vi "MWT_labview_final2.vi"() -> ()   [LabVIEW 2019]
uses:
  <vilib>/BLE/type_def/connection_status_bundle.ctl
  <vilib>/BLE/type_def/address_type.ctl
  <vilib>/BLE/ble_functions/ble_write_by_service_characteristic_uint8array.vi
panel:
  out "Omega0":dbl(graph)
  out "Omega0":dbl
  out "characteristic value":u8[](array[numeric])
  in  "transmission inteveral (Seconds)":u8[](array[numeric]) format="%02x"
  out "Omega4":dbl(graph)
  out "Omega4":dbl
  out "Omega1":dbl(graph)
  out "Omega1":dbl
  out "Omega3":dbl(graph)
  out "Omega3":dbl
  in  "stop":bool
  out "Reading data":bool
  out "Connected":bool
  out "Device Name":string
  out "Handle table":string[][](array[string])
  out "Connection Status":T1={"MAC Address"="", "cnx handle"=0, "cnx flags"=0, "Address Type"=125, "Connection Interval (ms)"=125, "Timeout(ms)"=125, "Latency"=0, "bonding handle"=0} {"Address Type" items=["Public", "Random"]}
  out "Scanning":bool
  in  "COM Bluegiga in":refnum<visa-resource-name>="COM13"
  out "Devices":string[][](array[string])
  out "BLED112 Dongle Info":string
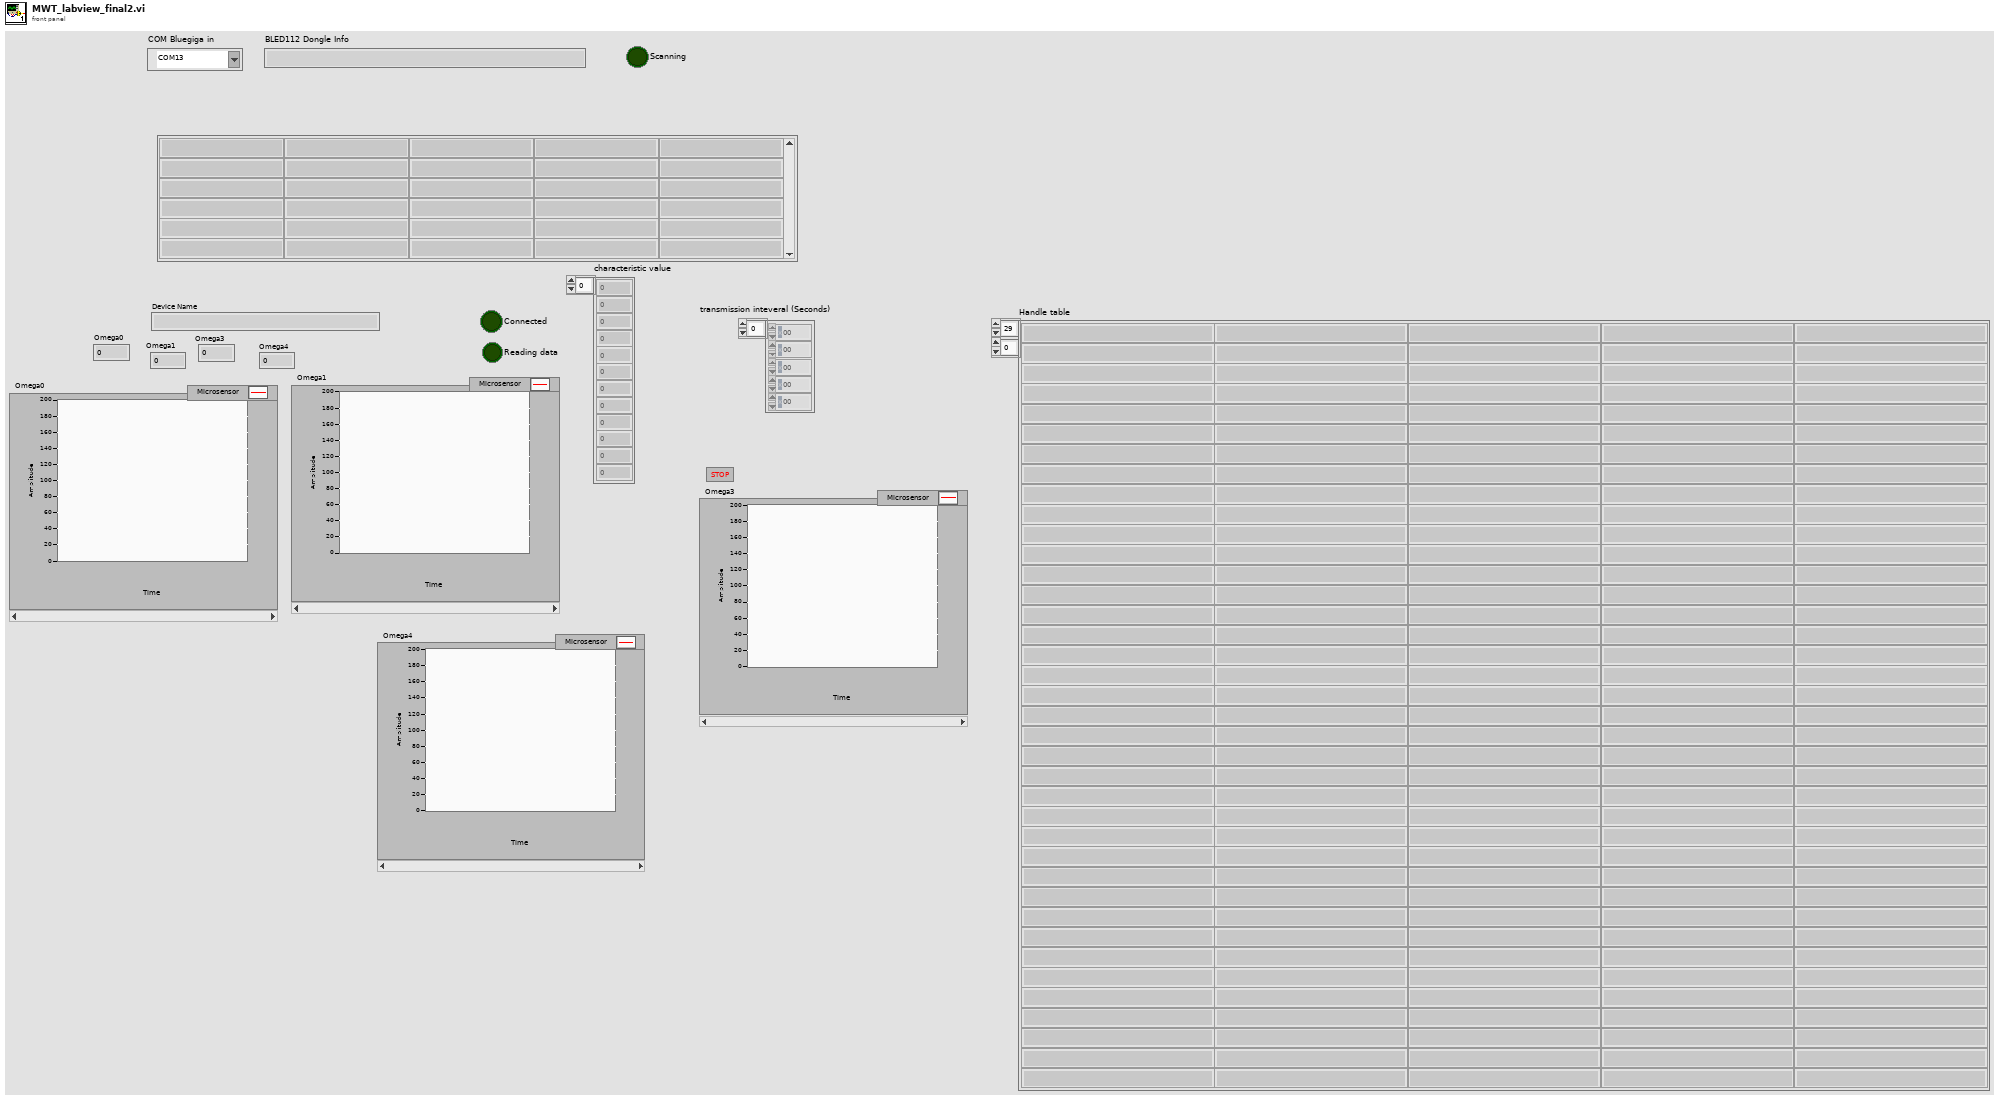
[diagram p1: front panel]
types:
  T1 = typedef "connection_status_bundle.ctl" = cluster{"MAC Address":string, "cnx handle":u8, "cnx flags":u8, "Address Type":T2, "Connection Interval (ms)":u16, "Timeout(ms)":u16, "Latency":u16, "bonding handle":u8}
  T2 = typedef "address_type.ctl" = u8
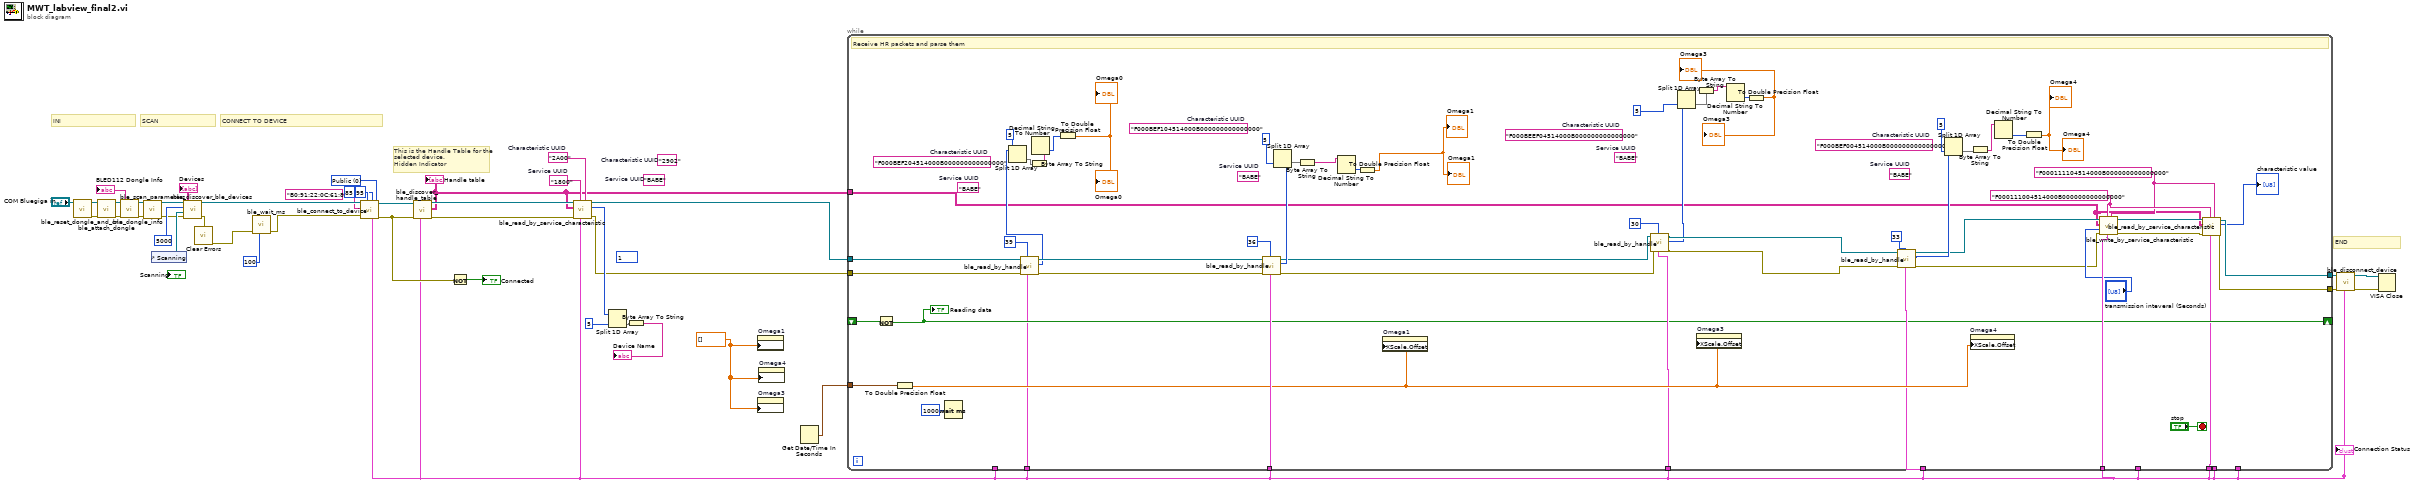
[diagram p0: block diagram]
diagram:
  w14 = T2 0 items=["Public", "Random"] ("Address Type")
  w12 = dbl[] [] ("History Data")
  (unwired) "2902"  # Characteristic UUID
  (unwired) "BABE"  # Service UUID
  (unwired) u16 1 ("Value(16bit)")
  w21 = "2A00"  # Characteristic UUID
  w22 = "1800"  # Service UUID
  # "END"
  # "This is the Handle Table for the\nselected device. \nHidden Indicator"
  # "CONNECT TO DEVICE"
  # "SCAN"
  # "INI"
  n1 = call <vilib>:"ble_reset_dongle_and_cnx.vi"("COM Bluegiga in"="COM Bluegiga in") -> ("error out"=w33:errorcluster, "COM Bluegiga out"=w31:refnum<visa-resource-name>)  [unwired: 9 in]
  n2 = call <vilib>:"ble_attach_dongle.vi"("error in (no error)"=w33, "COM Bluegiga in"=w31) -> ("error out"=w35:errorcluster, "COM Bluegiga out"=w34:refnum<visa-resource-name>)  [unwired: 8 in]
  n3 = call <vilib>:"ble_dongle_info.vi"("error in (no error)"=w35, "COM Bluegiga in"=w34) -> ("error out"=w38:errorcluster, "info"=→"BLED112 Dongle Info":string, "COM Bluegiga out"=w39:refnum<visa-resource-name>)  [unwired: 7 in]
  n4 = call <vilib>:"ble_scan_parameters.vi"("error in (no error)"=w38, "COM Bluegiga in"=w39) -> ("error out"=w36:errorcluster, "COM Bluegiga out"=w37:refnum<visa-resource-name>)  [unwired: 7 in, 1 out]
  n5 = control-ref of="Scanning"() -> (w40:refnum<vi>)
  n6 = call <vilib>:"ble_discover_ble_devices.vi"("error in (no error)"=w36, "LED ref"=w40, "Scan Duration (10000ms)"=u32 5000, "COM Bluegiga in"=w37) -> ("error out"=w29:errorcluster, "Devices"=→"Devices":string[][], "COM Bluegiga out"=w15:refnum<visa-resource-name>)  [unwired: 5 in]
  n7 = call <vilib>:"Clear Errors.vi"("error in (no error)"=w29) -> ("error out"=w18:errorcluster)  [unwired: 5 in, 1 out]
  n8 = call <vilib>:"ble_wait_ms.vi"("milliseconds to wait (100)"=u32 100, "error in (no error)"=w18) -> ("error out"=w17:errorcluster)  [unwired: 9 in]
  n9 = call <vilib>:"ble_connect_to_device.vi"("Address Type"=w14, "Connection Interval Max (95ms)"=u16 95, "Connection Interval Min (75ms)"=u16 85, "error in (no error)"=w17, "MAC Address"="B0:91:22:0C:61:84", "COM Bluegiga in"=w15) -> ("error out"=w23:errorcluster, "COM Bluegiga out"=w30:refnum<visa-resource-name>, "Connection Status"=w2:T1)  [unwired: 3 in]
  "Connection Status" <- w2
  n10 = call <vilib>:"ble_discover_handle_table.vi"("Connection Status"=w2, "error in (no error)"=w23, "COM Bluegiga in"=w30) -> ("error out"=w28:errorcluster, "Handle table"=w1:string[][], "COM Bluegiga out"=w27:refnum<visa-resource-name>)  [unwired: 6 in]
  "Handle table" <- w1
  n11 = Not(x=w23) -> (.not. x?=→"Connected":bool)
  n12 = call <vilib>:"ble_read_by_service_characteristic.vi"("Characteristic UUID"=w21, "Connection Status"=w2, "Service UUID"=w22, "error in (no error)"=w28, "Handle table"=w1, "COM Bluegiga in"=w27) -> ("error out"=w5:errorcluster, "characteristic value"=w20:u8[], "COM Bluegiga out"=w6:refnum<visa-resource-name>)  [unwired: 3 in]
  n13 = Split 1D Array(array=w20, index=5) -> (second subarray=w19:u8[])  [unwired: 1 out]
  n14 = Byte Array To String(unsigned byte array=w19) -> (string=→"Device Name":string)
  n15 = property on="Omega1" class="WFChart (strict)"("History Data"=w12) -> ()  [unwired: 2 in, 2 out]
  n16 = property on="Omega3" class="WFChart (strict)"("History Data"=w12) -> ()  [unwired: 2 in, 2 out]
  n17 = property on="Omega4" class="WFChart (strict)"("History Data"=w12) -> ()  [unwired: 2 in, 2 out]
  n18 = Get Date/Time In Seconds() -> (seconds since 1Jan1904=w9:timestamp)
  n19 = while {
    shift-right: [w72] -> _
    shift-left: _ -> [w101]
    tunnel: w2 -> [w76]
    tunnel: w2 -> [w92]
    tunnel: w2 -> [_]
    tunnel: w2 -> [w74]
    tunnel: w9 -> [w82]
    tunnel: w2 -> [_]
    tunnel: w2 -> [w80]
    tunnel: w6 -> [w68]
    tunnel: w5 -> [w67]
    tunnel: w2 -> [w66]
    tunnel: w2 -> [_]
    tunnel: w2 -> [_]
    tunnel: [w54] -> w4
    tunnel: [w53] -> w3
    tunnel: w2 -> [w49]
    tunnel: w1 -> [w48]
    stop <- "stop" stop-if-true
    w51 = "F000111004514000B000000000000000" ("Service UUID")
    w50 = "F000111104514000B000000000000000" ("Characteristic UUID")
    (unwired) "F000BEF004514000B000000000000000"  # Characteristic UUID
    (unwired) "BABE"  # Service UUID
    (unwired) "F000BEF204514000B000000000000000"  # Characteristic UUID
    (unwired) "BABE"  # Service UUID
    (unwired) "F000BEF104514000B000000000000000"  # Characteristic UUID
    (unwired) "BABE"  # Service UUID
    (unwired) "F000BEEF04514000B000000000000000"  # Characteristic UUID
    (unwired) "BABE"  # Service UUID
    # "Receive HR packets and parse them"
    n20 = Not(x=w101) -> (.not. x?=w72:bool)
    "Reading data" <- w72
    n21 = To Double Precision Float(number=w82) -> (double precision float=w83:dbl)
    n22 = Wait (ms)(milliseconds to wait=u32 1000) -> ()  [unwired: 1 out]
    n23 = call <vilib>:"ble_read_by_handle.vi"("Connection Status"=w66, "Handle"=u16 39, "error in (no error)"=w67, "COM Bluegiga in"=w68) -> ("error out"=w70:errorcluster, "characteristic value"=w65:u8[], "COM Bluegiga out"=w71:refnum<visa-resource-name>)  [unwired: 5 in]
    n24 = Split 1D Array(array=w65, index=5) -> (second subarray=w57:u8[])  [unwired: 1 out]
    n25 = Byte Array To String(unsigned byte array=w57) -> (string=w90:string)
    n26 = Decimal String To Number(string=w90) -> (number=w89:i32)  [unwired: 2 in, 1 out]
    n27 = To Double Precision Float(number=w89) -> (double precision float=→"Omega0" →"Omega0":dbl)
    n28 = call <vilib>:"ble_read_by_handle.vi"("Connection Status"=w92, "Handle"=u16 36, "error in (no error)"=w70, "COM Bluegiga in"=w71) -> ("error out"=w77:errorcluster, "characteristic value"=w93:u8[], "COM Bluegiga out"=w78:refnum<visa-resource-name>)  [unwired: 5 in]
    n29 = Split 1D Array(array=w93, index=5) -> (second subarray=w94:u8[])  [unwired: 1 out]
    n30 = Byte Array To String(unsigned byte array=w94) -> (string=w46:string)
    n31 = Decimal String To Number(string=w46) -> (number=w47:i32)  [unwired: 2 in, 1 out]
    n32 = To Double Precision Float(number=w47) -> (double precision float=→"Omega1" →"Omega1":dbl)
    n33 = property on="Omega1" class="WFChart (strict)"("XScale.Offset"=w83) -> ()  [unwired: 2 in, 2 out]
    n34 = call <vilib>:"ble_read_by_handle.vi"("Connection Status"=w76, "Handle"=u16 30, "error in (no error)"=w77, "COM Bluegiga in"=w78) -> ("error out"=w63:errorcluster, "characteristic value"=w62:u8[], "COM Bluegiga out"=w64:refnum<visa-resource-name>)  [unwired: 5 in]
    n35 = Split 1D Array(array=w62, index=5) -> (second subarray=w99:u8[])  [unwired: 1 out]
    n36 = property on="Omega3" class="WFChart (strict)"("XScale.Offset"=w83) -> ()  [unwired: 2 in, 2 out]
    n37 = Byte Array To String(unsigned byte array=w99) -> (string=w98:string)
    n38 = Decimal String To Number(string=w98) -> (number=w97:i32)  [unwired: 2 in, 1 out]
    n39 = To Double Precision Float(number=w97) -> (double precision float=→"Omega3" →"Omega3":dbl)
    n40 = call <vilib>:"ble_read_by_handle.vi"("Connection Status"=w74, "Handle"=u16 33, "error in (no error)"=w63, "COM Bluegiga in"=w64) -> ("error out"=w58:errorcluster, "characteristic value"=w60:u8[], "COM Bluegiga out"=w59:refnum<visa-resource-name>)  [unwired: 5 in]
    n41 = Split 1D Array(array=w60, index=5) -> (second subarray=w87:u8[])  [unwired: 1 out]
    n42 = property on="Omega4" class="WFChart (strict)"("XScale.Offset"=w83) -> ()  [unwired: 2 in, 2 out]
    n43 = Byte Array To String(unsigned byte array=w87) -> (string=w86:string)
    n44 = Decimal String To Number(string=w86) -> (number=w85:i32)  [unwired: 2 in, 1 out]
    n45 = To Double Precision Float(number=w85) -> (double precision float=→"Omega4" →"Omega4":dbl)
    n46 = call-poly <vilib>:"ble_write_by_service_characteristic.vi"("Characteristic UUID"=w50, "Connection Status"=w80, "Service UUID"=w51, "error in (no error)"=w58, "data"="transmission inteveral (Seconds)", "Handle table"=w48, "COM Bluegiga in"=w59) -> ("error out"=w55:errorcluster, "COM Bluegiga out"=w56:refnum<visa-resource-name>)  [unwired: 3 in]
    n47 = call <vilib>:"ble_read_by_service_characteristic.vi"("Characteristic UUID"=w50, "Connection Status"=w49, "Service UUID"=w51, "error in (no error)"=w55, "Handle table"=w48, "COM Bluegiga in"=w56) -> ("error out"=w53:errorcluster, "characteristic value"=→"characteristic value":u8[], "COM Bluegiga out"=w54:refnum<visa-resource-name>)  [unwired: 3 in]
  }
  n48 = call <vilib>:"ble_disconnect_device.vi"("Connection Status"=w2, "error in (no error)"=w3, "COM Bluegiga in"=w4) -> ("error out"=w10:errorcluster, "COM Bluegiga out"=w11:refnum<visa-resource-name>)  [unwired: 7 in]
  n49 = VISA Close(VISA resource name=w11, error in (no error)=w10) -> ()  [unwired: 1 out]
